vi "Request Database.vi"(8 "error in (no error)":errorcluster, 11 "TestCase in":refnum<class "Test DataBase.lvclass">) -> (0 "error out":errorcluster, 3 "TestCase out":refnum<class "Test DataBase.lvclass">)   [LabVIEW 2020, in "Test DataBase.lvclass"]
uses:
  Test DataBase.lvclass
  User Interface/User Interface.lvclass
  User Interface/User Interface.lvclass/User Interface.ctl
  <vilib>/addons/_JKI Toolkits/VI Tester/TestCase.llb/TestCase.lvclass
  C:/Program Files (x86)/National Instruments/LabVIEW 2020/vi.lib/addons/_JKI Toolkits/VI Tester/TestCase.llb/TestCase.lvclass
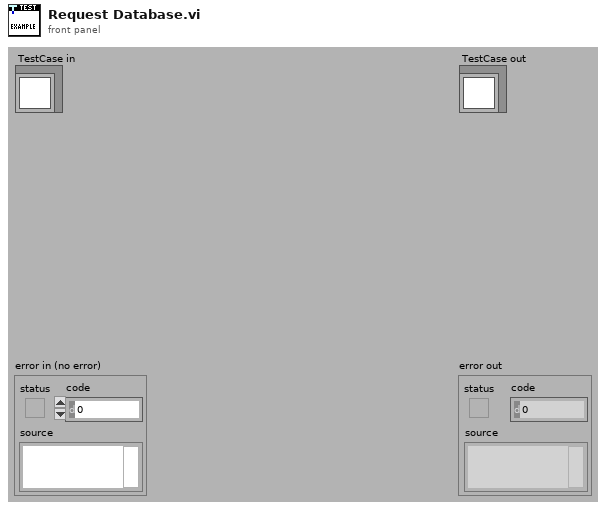
[diagram p1: front panel]
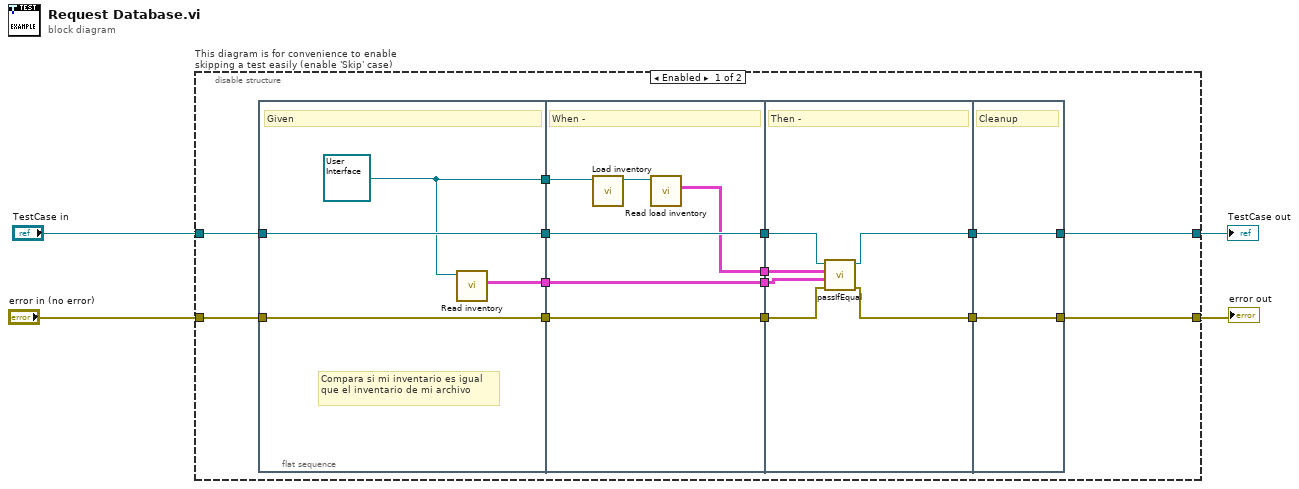
[diagram p0: block diagram]
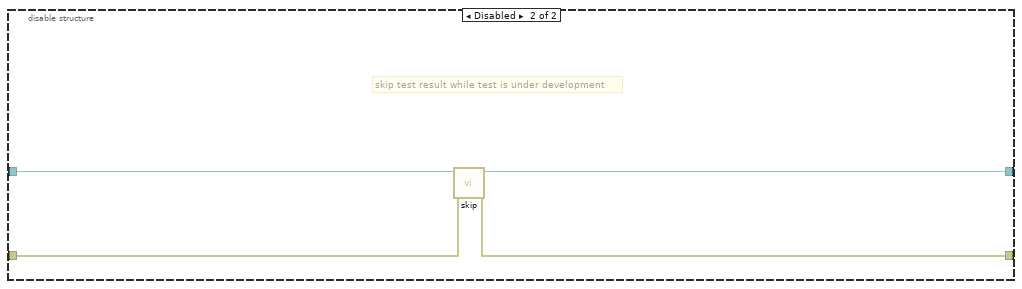
[diagram p2: hidden frame]
diagram:
  n1 = disable-structure "This diagram is for convenience to enable skipping a test easily (enable 'Skip' case)" shown="Enabled" {
    disable-tunnel: "TestCase in" -> [w12 w40]
    disable-tunnel: [w10 w38] -> w1
    disable-tunnel: [w9 w39] -> w3
    disable-tunnel: "error in (no error)" -> [w11 w37]
    frame Enabled {
      n2 = flat-sequence {
        tunnel: w11 -> [w21]
        tunnel: w12 -> [w22]
        tunnel: [w22] -> w18
        tunnel: [w21] -> w17
        tunnel: [w19] -> w7
        tunnel: [w20] -> w5
        tunnel: [w28] -> w16
        tunnel: [w27] -> w15
        tunnel: w18 -> [w28]
        tunnel: w17 -> [w27]
        tunnel: [w25] -> w8
        tunnel: w7 -> [w24]
        tunnel: [w23] -> w6
        tunnel: w5 -> [w23]
        tunnel: [w33] -> w14
        tunnel: [w31] -> w13
        tunnel: w16 -> [w34]
        tunnel: w15 -> [w32]
        tunnel: w8 -> [w30]
        tunnel: w6 -> [w29]
        tunnel: [w35] -> w9
        tunnel: [w36] -> w10
        tunnel: w14 -> [w36]
        tunnel: w13 -> [w35]
        frame #0 {
          w19 = refnum<class "User Interface.lvclass"> refnum ("User Interface.lvlib:User Interface.lvclass")
          # "Compara si mi inventario es igual que el inventario de mi archivo"
          # "Given"
          n3 = call "Read inventory.vi"("User Interface in"=w19) -> ("inventory"=w20:cluster{"String":string, "value":u32, bool}[][])  [unwired: 8 in, 2 out]
        }
        frame #1 {
          # "When -"
          n4 = call "Load inventory.vi"("User Interface in"=w24) -> ("User Interface out"=w26:refnum<class "User Interface.lvclass">)  [unwired: 9 in, 1 out]
          n5 = call "Read load inventory.vi"("User Interface in"=w26) -> ("load inventory"=w25:cluster{"String":string, "value":u32, bool}[][])  [unwired: 8 in, 2 out]
        }
        frame #2 {
          # "Then -"
          n6 = call-dynamic "passIfEqual.vi"("error in (no error)"=w32, "y"=w29, "x"=w30, "TestCase in"=w34) -> ("error out"=w31:errorcluster, "TestCase out"=w33:refnum<class "Test DataBase.lvclass">)  [unwired: 6 in]
        }
        frame #3 {
          # "Cleanup"
        }
      }
    }
    frame Disabled {
      # "skip test result while test is under development"
      n7 = call <vilib>:"skip.vi"("error in (no error)"=w37, "TestCase in"=w40) -> ("error out"=w39:errorcluster, "TestCase out"=w38:refnum<class "Test DataBase.lvclass">)  [unwired: 8 in]
    }
  }
  "error out" <- w3
  "TestCase out" <- w1
